vi "New.vi"(6 "Delimiters":T1={"Close"="}}", "Open"="{{"}, 8 "Error In":errorcluster, 11 "New Delimiters":T1) -> (0 "Error Out":errorcluster, 3 "Delimiter":refnum<class "Delimiter.lvclass">)   [LabVIEW 2018, in "Toolkit.lvlib" / "Nodes.lvlib" / "Delimiter.lvclass"]
doc: "Creates a new Set Delimiter node that represents a Mustache Set Delimiter tag in a parsed template."
uses:
  Delimiter.lvclass
  Type Definitions/Delimiters.ctl
  Delimiter.lvclass/Delimiter.ctl
  Toolkit.lvlib
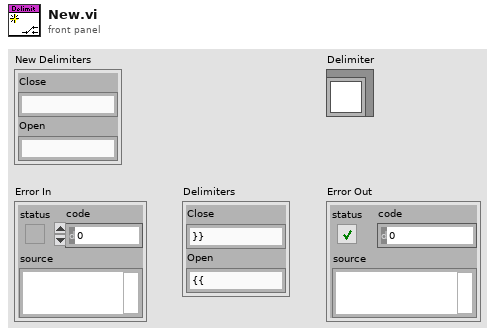
[diagram p1: front panel]
types:
  T1 = typedef "Toolkit.lvlib/Delimiters.ctl" = cluster{"Close":string, "Open":string}
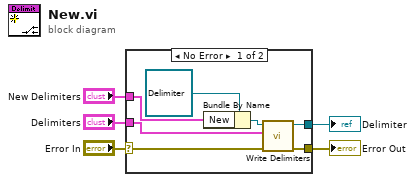
[diagram p0: block diagram]
diagram:
  n1 = case shown="No Error" "Error In" {
    selector: "Error In" -> [w8 w13]
    tunnel: "New Delimiters" -> [w11 _]
    tunnel: "Delimiters" -> [w9 _]
    tunnel: [w7 w13] -> w2
    tunnel: [w6 _] -> w1
    frame No Error {
      n2 = Bundle By Name(cluster=refnum<class "Delimiter.lvclass"> refnum ("Toolkit.lvlib:Nodes.lvlib:Delimiter.lvclass"), "New"=w11) -> (w10:refnum<class "Delimiter.lvclass">)
      n3 = call-dynamic "Write Delimiters.vi"("Error In"=w8, "Delimiters"=w9, "Node In"=w10) -> ("Error Out"=w7:errorcluster, "Node Out"=w6:refnum<class "Delimiter.lvclass">)  [unwired: 7 in]
    }
    frame Error {
    }
  }
  "Error Out" <- w2
  "Delimiter" <- w1
